vi "Image_Arithmetic.vi"() -> ()   [LabVIEW 2013]
uses:
  <vilib>/vision/NI_Vision_Development_Module.lvlib
panel:
  out "Image":T1(plugin-control)
  in  "Path 2":path
  in  "Enum":enum16{"ADD", "SUBTRACT", "MULTIPLY", "DIVIDE"}(ring)
  in  "Path":path
  in  "Boolean":bool
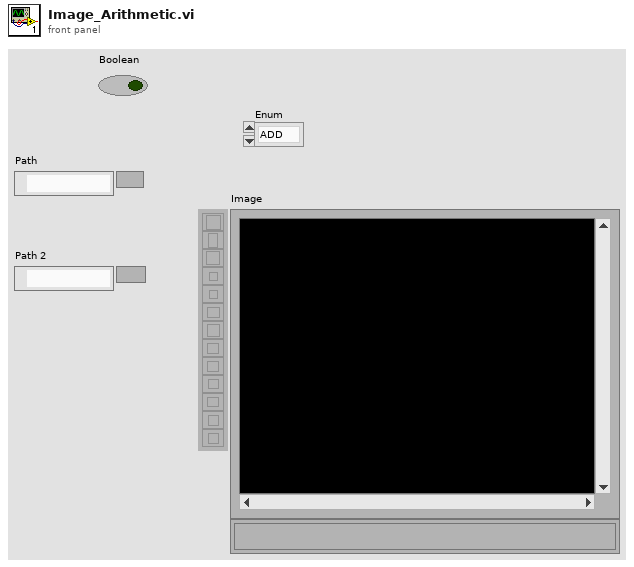
[diagram p1: front panel]
types:
  T1 = typedef "IMAQ Image.ctl" = refnum<image>
  T2 = typedef "Image Type" = u32
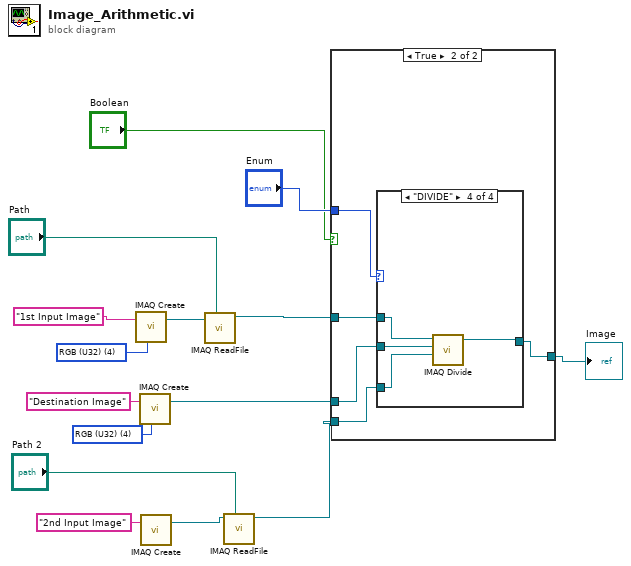
[diagram p0: block diagram]
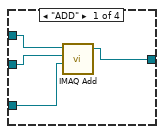
[diagram p3: hidden frame]
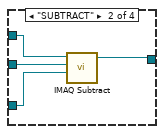
[diagram p4: hidden frame]
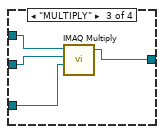
[diagram p5: hidden frame]
diagram:
  w1 = T2 4 items=["Grayscale (U8)", "Grayscale (I16)", "Grayscale (SGL)", "Complex (CSG)", "RGB (U32)", "HSL (U32)", "RGB (U64)", "Grayscale (U16)"] ("Image Type")
  w2 = T2 4 items=["Grayscale (U8)", "Grayscale (I16)", "Grayscale (SGL)", "Complex (CSG)", "RGB (U32)", "HSL (U32)", "RGB (U64)", "Grayscale (U16)"] ("Image Type")
  n1 = call "IMAQ Create"("Image Name"="1st Input Image", "Image Type"=w2) -> ("New Image"=w12:T1)  [unwired: 3 in, 1 out]
  n2 = call "IMAQ Create"("Image Name"="Destination Image", "Image Type"=w1) -> ("New Image"=w6:T1)  [unwired: 3 in, 1 out]
  n3 = call "IMAQ Create"("Image Name"="2nd Input Image") -> ("New Image"=w10:T1)  [unwired: 4 in, 1 out]
  n4 = call "IMAQ ReadFile"("File Path"="Path", "Image"=w12) -> ("Image Out"=w7:T1)  [unwired: 5 in, 4 out]
  n5 = call "IMAQ ReadFile"("File Path"="Path 2", "Image"=w10) -> ("Image Out"=w5:T1)  [unwired: 5 in, 4 out]
  n6 = case shown="True" "Boolean" {
    tunnel: "Enum" -> [_ w17]
    tunnel: w7 -> [_ w20]
    tunnel: w6 -> [_ w19]
    tunnel: w5 -> [_ w18]
    tunnel: [_ w16] -> w3
    frame False {
    }
    frame True {
      n7 = case shown="\"DIVIDE\"" w17 {
        tunnel: w20 -> [w24 w28 w32 w36]
        tunnel: w19 -> [w23 w27 w31 w35]
        tunnel: w18 -> [w22 w26 w30 w34]
        tunnel: [w21 w25 w29 w33] -> w16
        frame "ADD" {
          n8 = call "IMAQ Add"("Image Src A"=w24, "Image Dst"=w23, "Image Src B"=w22) -> ("Image Dst Out"=w21:T1)  [unwired: 4 in, 1 out]
        }
        frame "SUBTRACT" {
          n9 = call "IMAQ Subtract"("Image Src A"=w28, "Image Dst"=w27, "Image Src B"=w26) -> ("Image Dst Out"=w25:T1)  [unwired: 4 in, 1 out]
        }
        frame "MULTIPLY" {
          n10 = call "IMAQ Multiply"("Image Src A"=w32, "Image Dst"=w31, "Image Src B"=w30) -> ("Image Dst Out"=w29:T1)  [unwired: 4 in, 1 out]
        }
        frame "DIVIDE" {
          n11 = call "IMAQ Divide"("Image Src A"=w36, "Image Dst"=w35, "Image Src B"=w34) -> ("Image Dst Out"=w33:T1)  [unwired: 4 in, 1 out]
        }
      }
    }
  }
  "Image" <- w3
